vi "LightSetup.vi"(11 "PWMPeriodMultiplier":T4 items=["1X"=0, "2X"=1, "4X"=3]) -> (3 "Swag Light Ref cluster":T3)   [LabVIEW 2015]
doc: "This vi will take an array of ports, initalize the light and default values, and output the array of refrences to the newly initalized lights."
uses:
  <vilib>/Rock Robotics/WPI/PWM/WPI_PWMPeriodMultiplier.ctl
  <vilib>/Rock Robotics/WPI/PWM/WPI_PWMDeviceRef.ctl
  <vilib>/Rock Robotics/SystemInterfaces/DIO/FPGA_DIOPWMChannel.ctl
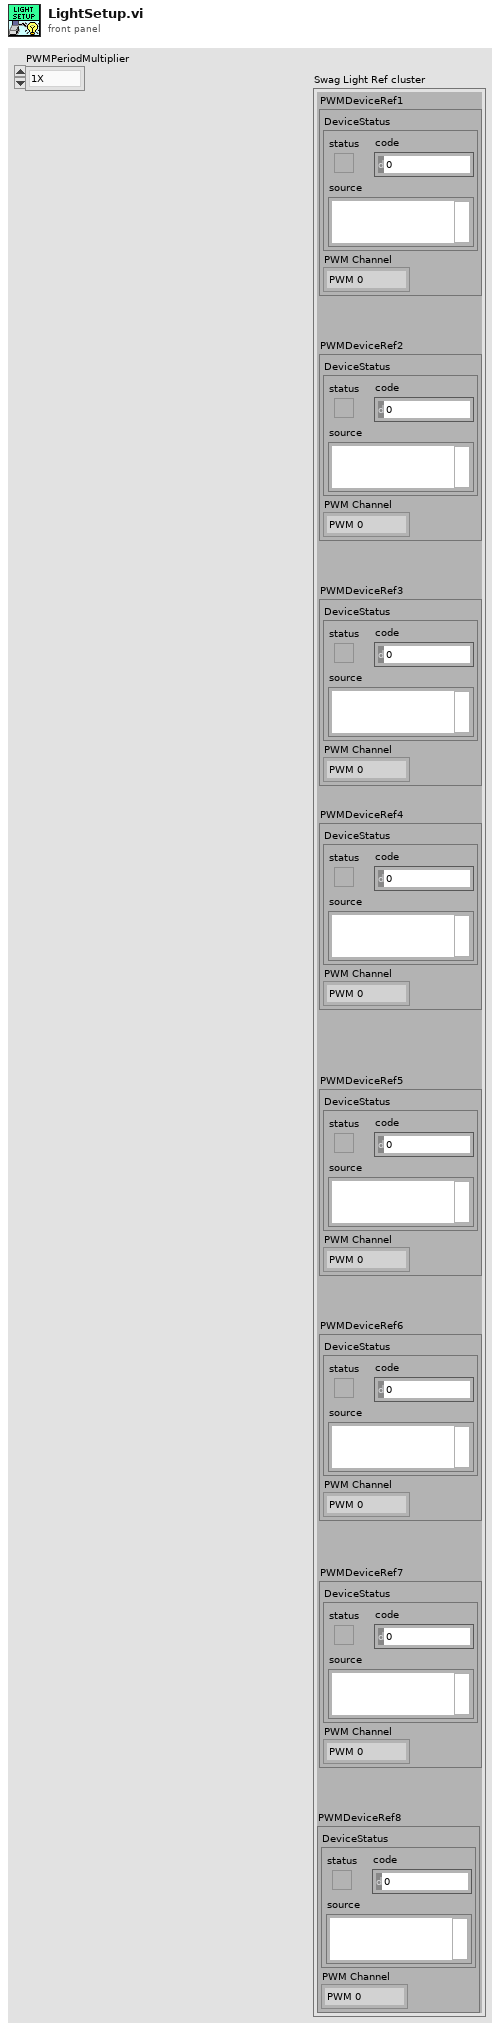
[diagram p1: front panel]
types:
  T1 = typedef "WPI_PWMDeviceRef.ctl" = cluster{"DeviceStatus":errorcluster, "PWM Channel":T2}
  T2 = typedef "FPGA_DIOPWMChannel.ctl" = enum8{"PWM 0", "PWM 1", "PWM 2", "PWM 3", "PWM 4", "PWM 5", "PWM 6", "PWM 7", "PWM 8", "PWM 9", "PWM MXP 0", "PWM MXP 1", "PWM MXP 2", "PWM MXP 3", "PWM MXP 4", "PWM MXP 5", "PWM MXP 6", "PWM MXP 7", "PWM MXP 8", "PWM MXP 9", "Invalid"}
  T3 = cluster{"PWMDeviceRef1":T1, "PWMDeviceRef2":T1, "PWMDeviceRef3":T1, "PWMDeviceRef4":T1, "PWMDeviceRef5":T1, "PWMDeviceRef6":T1, "PWMDeviceRef7":T1, "PWMDeviceRef8":T1}
  T4 = typedef "WPI_PWMPeriodMultiplier.ctl" = u8
  T5 = cluster{"PWMDeviceRef":T1, "PWMDeviceRef":T1, "PWMDeviceRef":T1, "PWMDeviceRef":T1, "PWMDeviceRef":T1, "PWMDeviceRef":T1, "PWMDeviceRef":T1, "PWMDeviceRef":T1}
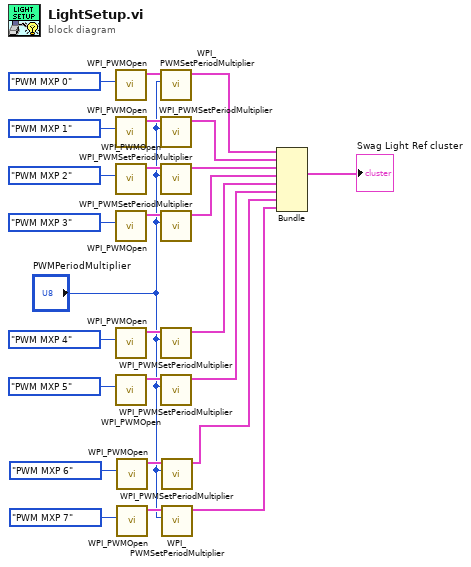
[diagram p0: block diagram]
diagram:
  n1 = call <vilib>:"WPI_PWMOpen.vi"("PWM Channel"=FPGA_DIOPWMChannel."PWM MXP 0") -> ("PWMDeviceRef"=w15:T1)  [unwired: 9 in, 1 out]
  n2 = call <vilib>:"WPI_PWMOpen.vi"("PWM Channel"=FPGA_DIOPWMChannel."PWM MXP 1") -> ("PWMDeviceRef"=w16:T1)  [unwired: 9 in, 1 out]
  n3 = call <vilib>:"WPI_PWMOpen.vi"("PWM Channel"=FPGA_DIOPWMChannel."PWM MXP 2") -> ("PWMDeviceRef"=w17:T1)  [unwired: 9 in, 1 out]
  n4 = call <vilib>:"WPI_PWMOpen.vi"("PWM Channel"=FPGA_DIOPWMChannel."PWM MXP 3") -> ("PWMDeviceRef"=w18:T1)  [unwired: 9 in, 1 out]
  n5 = call <vilib>:"WPI_PWMOpen.vi"("PWM Channel"=FPGA_DIOPWMChannel."PWM MXP 4") -> ("PWMDeviceRef"=w19:T1)  [unwired: 9 in, 1 out]
  n6 = call <vilib>:"WPI_PWMOpen.vi"("PWM Channel"=FPGA_DIOPWMChannel."PWM MXP 5") -> ("PWMDeviceRef"=w20:T1)  [unwired: 9 in, 1 out]
  n7 = call <vilib>:"WPI_PWMOpen.vi"("PWM Channel"=FPGA_DIOPWMChannel."PWM MXP 6") -> ("PWMDeviceRef"=w4:T1)  [unwired: 9 in, 1 out]
  n8 = call <vilib>:"WPI_PWMOpen.vi"("PWM Channel"=FPGA_DIOPWMChannel."PWM MXP 7") -> ("PWMDeviceRef"=w5:T1)  [unwired: 9 in, 1 out]
  n9 = call <vilib>:"WPI_PWMSetPeriodMultiplier.vi"("PWMPeriodMultiplier"="PWMPeriodMultiplier", "PWMDeviceRef"=w15) -> ("PWMDeviceRef"=w14:T1)  [unwired: 8 in, 1 out]
  n10 = call <vilib>:"WPI_PWMSetPeriodMultiplier.vi"("PWMPeriodMultiplier"="PWMPeriodMultiplier", "PWMDeviceRef"=w16) -> ("PWMDeviceRef"=w13:T1)  [unwired: 8 in, 1 out]
  n11 = call <vilib>:"WPI_PWMSetPeriodMultiplier.vi"("PWMPeriodMultiplier"="PWMPeriodMultiplier", "PWMDeviceRef"=w17) -> ("PWMDeviceRef"=w12:T1)  [unwired: 8 in, 1 out]
  n12 = call <vilib>:"WPI_PWMSetPeriodMultiplier.vi"("PWMPeriodMultiplier"="PWMPeriodMultiplier", "PWMDeviceRef"=w18) -> ("PWMDeviceRef"=w11:T1)  [unwired: 8 in, 1 out]
  n13 = call <vilib>:"WPI_PWMSetPeriodMultiplier.vi"("PWMPeriodMultiplier"="PWMPeriodMultiplier", "PWMDeviceRef"=w19) -> ("PWMDeviceRef"=w10:T1)  [unwired: 8 in, 1 out]
  n14 = call <vilib>:"WPI_PWMSetPeriodMultiplier.vi"("PWMPeriodMultiplier"="PWMPeriodMultiplier", "PWMDeviceRef"=w20) -> ("PWMDeviceRef"=w9:T1)  [unwired: 8 in, 1 out]
  n15 = call <vilib>:"WPI_PWMSetPeriodMultiplier.vi"("PWMPeriodMultiplier"="PWMPeriodMultiplier", "PWMDeviceRef"=w4) -> ("PWMDeviceRef"=w2:T1)  [unwired: 8 in, 1 out]
  n16 = call <vilib>:"WPI_PWMSetPeriodMultiplier.vi"("PWMPeriodMultiplier"="PWMPeriodMultiplier", "PWMDeviceRef"=w5) -> ("PWMDeviceRef"=w1:T1)  [unwired: 8 in, 1 out]
  n17 = Bundle("PWMDeviceRef"=w14, "PWMDeviceRef"=w13, "PWMDeviceRef"=w12, "PWMDeviceRef"=w11, "PWMDeviceRef"=w10, "PWMDeviceRef"=w9, "PWMDeviceRef"=w2, "PWMDeviceRef"=w1) -> (→"Swag Light Ref cluster":T5)  [unwired: 1 in]
